vi "Forces (SubVI).vi"(1 "Data":dbl[][](array[numeric]), 3 "act_b":dbl[](array[numeric]), 5 "Pdin [Pa], Patm [Pa], Temp [K], airflow velocity [m/s]":T8, 7 "AoA_pitch [rad], AoA_yaw [rad], Stream direction [rad]":T5, 9 "Vehicle Parameters":T2, 12 "i, sim_running, t[s], dt[s]":T3, 13 "V(i) [m/s] NWU, latd(i) [rad], lon(i) [rad], height(i) [m]":T7, 14 "Rotation":T1) -> (4 "M_alpha [rad/s^2], M_beta [rad/s^2]":T4, 6 "acc [m/s^2]":dbl[](array[numeric]), 10 "FE_b [N], FG [N], FA [N], Fco[N]":T6, 15 "FE [N]":dbl[](array[numeric]))   [LabVIEW 2017]
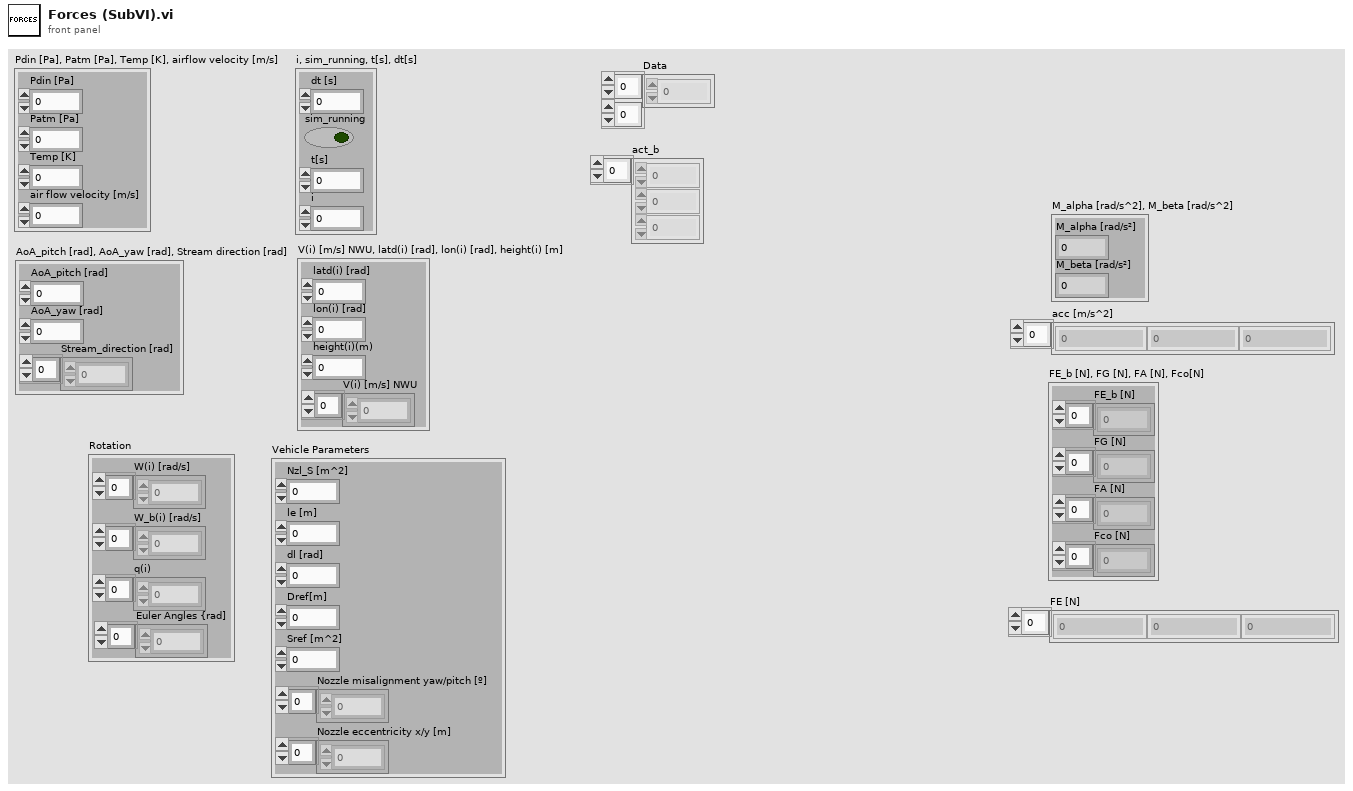
[diagram p1: front panel]
types:
  T1 = cluster{"W(i) [rad/s]":dbl[], "W_b(i) [rad/s]":dbl[], "q(i)":dbl[], "Euler Angles {rad]":dbl[]}
  T2 = cluster{"Nzl_S [m^2]":dbl, "le [m]":dbl, "dl [rad]":dbl, "Dref[m]":dbl, "Sref [m^2]":dbl, "Nozzle misalignment yaw/pitch [º]":dbl[], "Nozzle eccentricity x/y [m]":dbl[]}
  T3 = cluster{"dt [s]":dbl, "sim_running":bool, "t[s]":dbl, "i":i32}
  T4 = cluster{"M_alpha [rad/s²]":dbl, "M_beta [rad/s²]":dbl}
  T5 = cluster{"AoA_pitch [rad]":dbl, "AoA_yaw [rad]":dbl, "Stream_direction [rad]":dbl[]}
  T6 = cluster{"FE_b [N]":dbl[], "FG [N]":dbl[], "FA [N]":dbl[], "Fco [N]":dbl[]}
  T7 = cluster{"latd(i) [rad]":dbl, "lon(i) [rad]":dbl, "height(i)(m)":dbl, "V(i) [m/s] NWU":dbl[]}
  T8 = cluster{"Pdin [Pa]":dbl, "Patm [Pa]":dbl, "Temp [K]":dbl, "air flow velocity [m/s]":dbl}
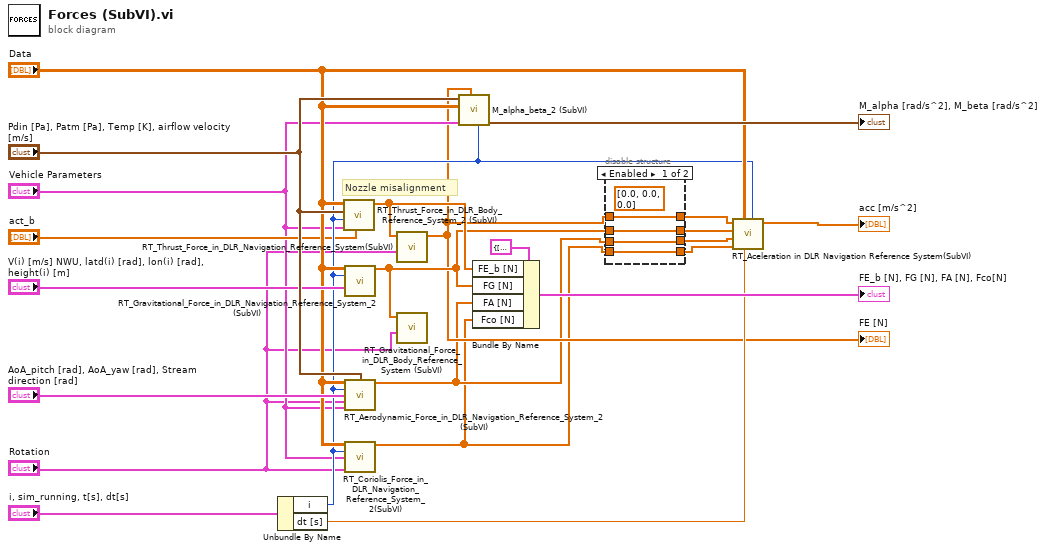
[diagram p0: block diagram]
diagram:
  # "Nozzle misalignment"
  n1 = Unbundle By Name("i, sim_running, t[s], dt[s]") -> ("i"=w13:i32, "dt [s]"=w20:dbl)
  n2 = call "RT_Thrust_Force_in_DLR_Body_Reference_System_2 (SubVI).vi"("Act_b(i)"="act_b", "Vehicle Parameters"="Vehicle Parameters", "i"=w13, "cluster"="Pdin [Pa], Patm [Pa], Temp [K], airflow velocity [m/s]", "Data"="Data") -> ("FE_b"=w14:dbl[])  [unwired: 6 in]
  n3 = call "RT_Gravitational_Force_in_DLR_Navigation_Reference_System_2 (SubVI).vi"("Data"="Data", "i"=w13, "input cluster"="V(i) [m/s] NWU, latd(i) [rad], lon(i) [rad], height(i) [m]") -> ("FG_d"=w8:dbl[])  [unwired: 11 in, 1 out]
  n4 = call "RT_Aerodynamic_Force_in_DLR_Navigation_Reference_System_2 (SubVI).vi"("Data"="Data", "input cluster 3"="Pdin [Pa], Patm [Pa], Temp [K], airflow velocity [m/s]", "i"=w13, "output cluster"="AoA_pitch [rad], AoA_yaw [rad], Stream direction [rad]", "Rotation"="Rotation", "Vehicle Parameters"="Vehicle Parameters") -> ("FA"=w4:dbl[])  [unwired: 8 in, 1 out]
  n5 = call "RT_Coriolis_Force_in_DLR_Navigation_Reference_System_2(SubVI).vi"("Data"="Data", "i"=w13, "Vehicle Parameters"="Vehicle Parameters", "Rotation"="Rotation") -> ("Fco (N)"=w2:dbl[])  [unwired: 11 in]
  n6 = call "RT_Thrust_Force_in_DLR_Navigation_Reference_System(SubVI).vi"("Rotation"="Rotation", "FE_b"=w14) -> ("FE"=w6:dbl[])  [unwired: 8 in]
  "FE [N]" <- w6
  n7 = call "RT_Gravitational_Force_in_DLR_Body_Reference_System (SubVI).vi"("Rotation"="Rotation", "FG_d"=w8) -> ()  [unwired: 9 in, 1 out]
  n8 = call "M_alpha_beta_2 (SubVI).vi"("i"=w13, "FE [N]"=w6, "Vehicle Parameters"="Vehicle Parameters", "Data"="Data", "cluster"="Pdin [Pa], Patm [Pa], Temp [K], airflow velocity [m/s]") -> ("output cluster"=→"M_alpha [rad/s^2], M_beta [rad/s^2]":T4)  [unwired: 4 in, 2 out]
  n9 = Bundle By Name(cluster=T6 {"FE_b [N]"=[], "FG [N]"=[], "FA [N]"=[], "Fco [N]"=[]} ("output cluster 2"), "FE_b [N]"=w14, "FG [N]"=w8, "FA [N]"=w4, "Fco [N]"=w2) -> (→"FE_b [N], FG [N], FA [N], Fco[N]":T6)
  n10 = disable-structure shown="Enabled" {
    disable-tunnel: w8 -> [w26 w31]
    disable-tunnel: [w26 w31] -> w7
    disable-tunnel: w6 -> [w25 w30]
    disable-tunnel: [w25 w30] -> w5
    disable-tunnel: w4 -> [w24 w29]
    disable-tunnel: [w24 w29] -> w3
    disable-tunnel: w2 -> [w27 w28]
    disable-tunnel: [w27 w28] -> w1
    frame Enabled {
      (unwired) dbl[] [0.0, 0.0, 0.0] ("FG_d")
    }
    frame Disabled {
    }
  }
  n11 = call "RT_Aceleration in DLR Navigation Reference System(SubVI).vi"("i"=w13, "dt(s)"=w20, "Data"="Data", "Fco (N)"=w1, "FA"=w3, "FG"=w7, "FE"=w5) -> ("acc"=→"acc [m/s^2]":dbl[])  [unwired: 4 in]
